vi "ex1_3b.vi"() -> ()   [LabVIEW 2017]
uses:
  <vilib>/measure/NI_MABase.lvlib
panel:
  out "Waveform Graph":waveform(dbl)(graph)={"t0"=timestamp(2.8 s since 1904-01-01), "dt"=0.0004, "Y"=array[1000 elements]}
  in  "Delay":dbl
  out "Frequency played":dbl=521.0
  in  "Sampling parameters":cluster{"Fs":dbl, "Samples":dbl}={"Fs"=2500.0, "Samples"=1000.0}
  in  "Phase":dbl
  in  "Amplitude":dbl=1.0
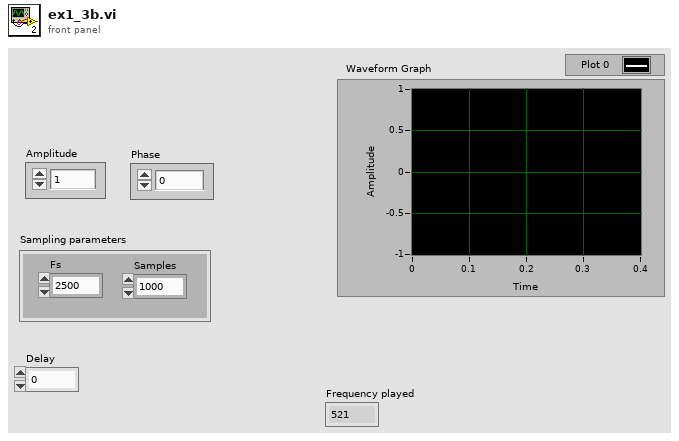
[diagram p1: front panel]
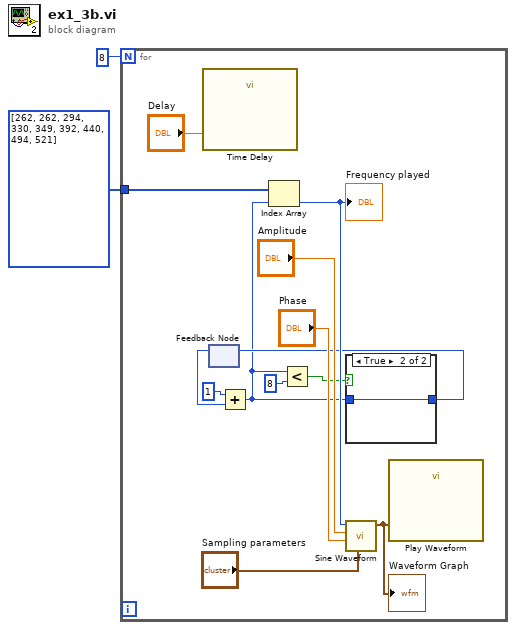
[diagram p0: block diagram]
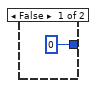
[diagram p2: hidden frame]
diagram:
  n1 = for {
    N: 8 -> [_]
    tunnel: i32[] [262, 262, 294, 330, 349, 392, 440, 494, 521] -> [w12]
    n2 = call "Time Delay"("Delay Time (s)"="Delay") -> ()  [unwired: 10 in, 1 out]
    n3 = feedback #1() -> (w6:i32)  [unwired: 1 in]
    n4 = Add(x=1, y=w6) -> (x+y=w5:i32)
    n5 = Index Array(array=w12, index=w5) -> (element=w11:i32)
    "Frequency played" <- w11
    n6 = Less?(x=w5, y=8) -> (x < y?=w9:bool)
    n7 = case shown="True" w9 {
      tunnel: w5 -> [_ w17]
      tunnel: [0 w17] -> w7
      frame False {
      }
      frame True {
      }
    }
    n8 = feedback-in #1(w7) -> ()
    n9 = call <vilib>:"Sine Waveform.vi"("sampling info"="Sampling parameters", "phase"="Phase", "amplitude"="Amplitude", "frequency"=w11) -> ("signal out"=w3:waveform(dbl))  [unwired: 6 in, 1 out]
    "Waveform Graph" <- w3
    n10 = call "Play Waveform"("Data"=w3) -> ()  [unwired: 18 in, 1 out]
  }
